vi "Raman multicurve no-readout fit vi.vi"() -> ()   [LabVIEW 2015]
uses:
  <vilib>/Utility/file.llb/Read From Spreadsheet File (DBL).vi
  <vilib>/Utility/file.llb/Read From Spreadsheet File (string).vi
  <vilib>/Utility/file.llb/Write To Spreadsheet File (string).vi
panel:
  out "estimated time to finish 2":i32
  in  "Seconds per curve":sgl=3.75
  out "estimated time to finish":i32
  in  "Correction\ncoefficient":i32
  in  "Polynomial baseline?":bool
  in  "Positive peaks only?":bool
  out "Fitting progress 2":i32(slide) scale=0.0..961.0
  out "Fitting progress":i32(slide) scale=0.0..3720.0
  out "Curve#":i32
  in  "ScanSize":i32=31
  in  "endX":dbl=1900.0
  in  "startX":dbl=1000.0
  in  "Initial Guess Coefficient":dbl[](array[numeric])=[1.0, 1.0, 1.0, 1.0, 1.0, 1.0, 1.0, 1.0, 1.0] format="%0.2f"
  in  "Save to file?":bool
  # "Make sure the path to PURE.DAT is correct in all\n\"LM model function\" formula files"
  # "To make minor adjustments for the fit.\nCAN BE CHANGED IN REAL TIME\nCAN BE NEGATIVE"
  # "1800-2700 for noise\n1000-1900 for sample"
  # "Disabled state = 1st order curve for base \nEnabled state =2nd order curve for base"
  # "= a1\n= a2\n= a3\n= a4"
  # "Fitting range:"
  # "Disabled state = negative peaks allowed\nEnabled state = only positive peaks"
  # "= a5\n= a6\n= poly coeff\n= line slope\n= line base"
  # "Note: No need to update LM model file any more"
  # "Disabled state = fit results not saved\nEnabled state = fit results saved to file"
  # "scan size 31"
  # "Estimated time to finish, min"
  # "scan size 61"
  # "Version 1.02\nAVM"
  # "dinamic time"
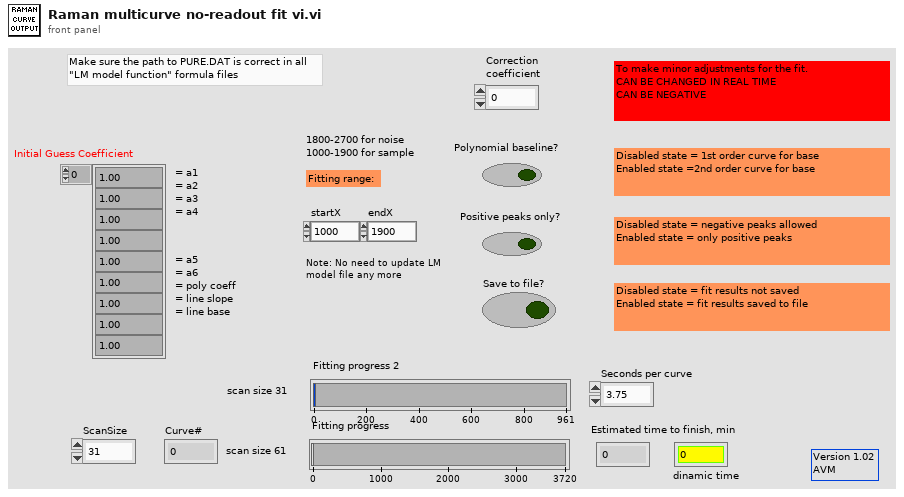
[diagram p1: front panel]
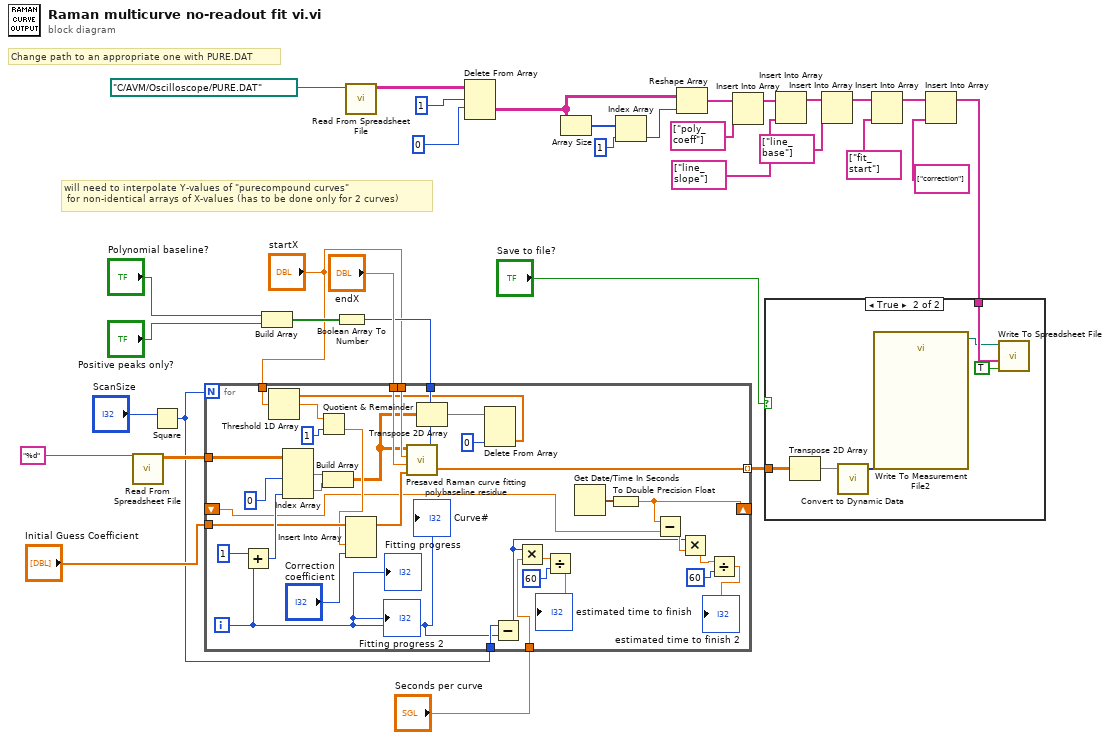
[diagram p0: block diagram]
diagram:
  # "Change path to an appropriate one with PURE.DAT"
  # "will need to interpolate Y-values of \"purecompound curves\"\n for non-identical arrays of X-values (has to be done only for 2 curves)"
  n1 = call-poly <vilib>:"Read From Spreadsheet File.vi"("format (%.3f)"="%d" ("format (%d)")) -> ("all rows"=w30:dbl[][])  [unwired: 6 in, 4 out]
  n2 = Square(x="ScanSize") -> (x^2=w2:i32)
  n3 = Build Array("Polynomial baseline?", "Positive peaks only?") -> (w13:bool[])
  n4 = Boolean Array To Number(Boolean array=w13) -> (number=w11:u32)
  n5 = for {
    N: w2 -> [_]
    tunnel: "endX" -> [w61]
    tunnel: "startX" -> [w62]
    tunnel: w30 -> [w63]
    tunnel: [w60] -> w24 mode=indexing
    tunnel: "Initial Guess Coefficient" -> [w57]
    tunnel: w11 -> [w56]
    tunnel: "startX" -> [w53]
    tunnel: w2 -> [w47]
    tunnel: "Seconds per curve" -> [w42]
    shift-right: [w35] -> _
    shift-left: _ -> [w34]
    i -> [w46]
    n6 = Add(x=1, y=w46) -> (x+y=w67:i32)
    n7 = Index Array(array=w63, index (col) #1=0 ("disabled index (col)"), index (col) #2=w67) -> (element #1=w66:dbl[], element #2=w65:dbl[])  [unwired: 2 in]
    n8 = Build Array(w66, w65) -> (w49:dbl[][])
    n9 = Transpose 2D Array(2D array=w49) -> (transposed array=w50:dbl[][])
    n10 = Delete From Array(array=w50, index (col)=0 ("disabled index (col)")) -> (deleted portion=w48:dbl[])  [unwired: 2 in, 1 out]
    n11 = Threshold 1D Array(2:w53, 3:w48) -> (0:w55:dbl)  [unwired: 1 in]
    n12 = Quotient & Remainder(x=w55, y=1) -> (floor(x/y)=w52:dbl)  [unwired: 1 out]
    n13 = Insert Into Array(array=w57, new element #1=w52, new element #2="Correction\ncoefficient") -> (w59:dbl[])  [unwired: 1 in]
    n14 = call "Presaved Raman curve fitting polybaseline residue.vi"("index"=w56, "Initial Guess Coefficient"=w59, "endX"=w61, "startX"=w62, "Selected data set per point"=w49) -> ("Coefficients"=w60:dbl[])
    n15 = Subtract(x=w47, y=w46) -> (x-y=w37:i32)
    n16 = Multiply(x=w37, y=w42) -> (x*y=w44:sgl)
    n17 = Divide(x=w44, y=60 ("disabled index (col)")) -> (x/y=→"estimated time to finish":sgl)
    n18 = Get Date/Time In Seconds() -> (seconds since 1Jan1904=w41:timestamp)
    n19 = To Double Precision Float(number=w41) -> (double precision float=w35:dbl)
    n20 = Subtract(x=w35, y=w34) -> (x-y=w38:dbl)
    n21 = Multiply(x=w37, y=w38) -> (x*y=w36:dbl)
    n22 = Divide(x=w36, y=60 ("disabled index (col)")) -> (x/y=→"estimated time to finish 2":dbl)
    "Curve#" <- w46
    "Fitting progress" <- w46
    "Fitting progress 2" <- w46
  }
  n23 = call-poly <vilib>:"Read From Spreadsheet File.vi"("file path (dialog if empty)"=path "C:/AVM/Oscilloscope/PURE.DAT") -> ("all rows"=w28:string[][])  [unwired: 6 in, 4 out]
  n24 = Delete From Array(array=w28, length=1 ("index (row)"), index (row)=0) -> (deleted portion=w21:string[][])  [unwired: 1 in, 1 out]
  n25 = Array Size(array=w21) -> (size(s)=w23:i32[])
  n26 = Index Array(array=w23, index=1) -> (element=w20:i32)
  n27 = Reshape Array(w21, w20) -> (w19:string[])
  n28 = Insert Into Array(array=w19, new element=string[] ["poly_coeff"] ("element")) -> (w17:string[])  [unwired: 1 in]
  n29 = Insert Into Array(array=w17, new element=string[] ["line_slope"] ("element")) -> (w6:string[])  [unwired: 1 in]
  n30 = Insert Into Array(array=w6, new element=string[] ["line_base"] ("element")) -> (w5:string[])  [unwired: 1 in]
  n31 = Insert Into Array(array=w5, new element=string[] ["fit_start"] ("element")) -> (w4:string[])  [unwired: 1 in]
  n32 = Insert Into Array(array=w4, new element=string[] ["correction"] ("element")) -> (w3:string[])  [unwired: 1 in]
  n33 = case shown="True" "Save to file?" {
    tunnel: w24 -> [_ w70]
    tunnel: w3 -> [_ w73]
    frame False {
    }
    frame True {
      n34 = Transpose 2D Array(2D array=w70) -> (transposed array=w69:dbl[][])
      n35 = call "Convert to Dynamic Data"("2D Array"=w69) -> ("Dynamic Data Type"=w74:dynamicdata)  [unwired: 3 in]
      n36 = call "Write To Measurement File2"("Signals"=w74) -> ("Filename Out"=w72:path)  [unwired: 16 in, 2 out]
      n37 = call-poly <vilib>:"Write To Spreadsheet File.vi"("append to file? (new file:F)"=TRUE, "1D data"=w73, "file path (dialog if empty)"=w72) -> ()  [unwired: 5 in, 1 out]
    }
  }
